vi "Compute Optimal Transition Time.vi"(8 "error in (no error)":errorcluster, 10 "optimum":T1, 11 "SV Function in":refnum<class "SV Function.lvclass">) -> (0 "error out":errorcluster, 2 "optimal transition time":dbl, 3 "SV Function out":refnum<class "SV Function.lvclass">)   [LabVIEW 2017, in "SV Function.lvclass"]
uses:
  <vilib>/addons/_NISVFA/_Generation/Signal Generation/SV Function/SV Function.lvclass
  C:/Program Files (x86)/National Instruments/LabVIEW 2017/vi.lib/addons/_NISVFA/_Generation/Signal Generation/SV Signal/SV Signal.lvclass
  <vilib>/addons/_NISVFA/_Generation/subVIs/sv_Optimum Location.ctl
  <vilib>/addons/_NISVFA/_Generation/Signal Generation/SV Signal/sv_Signal State Attribute.ctl
  <vilib>/addons/_NISVFA/_Generation/Signal Generation/SV Function/SV Function.lvclass/SV Function.ctl
  <vilib>/addons/_NISVFA/_Generation/Signal Generation/SV Signal/Read Sample Rate.vi
  <vilib>/addons/_NISVFA/_Generation/Signal Generation/SV Signal/SV Signal.lvclass
  <vilib>/addons/_NISVFA/_Generation/SoundVib_Generation.lvlib
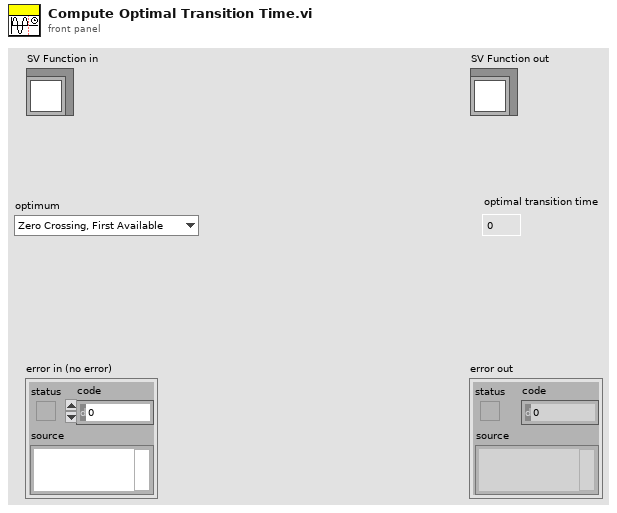
[diagram p1: front panel]
types:
  T1 = typedef "SoundVib_Generation.lvlib/sv_Optimum Location.ctl" = enum16{"Zero Crossing, First Available", "Zero Crossing, Positive Slope", "Zero Crossing, Negative Slope", "Peak or Valley", "Peak", "Valley"}
  T2 = typedef "SV Signal.lvclass/sv_Signal State Attribute.ctl" = string
  T3 = typedef "SV Signal.lvclass/sv_System Timing Model.ctl" = i64
  T4 = typedef "SV Signal.lvclass/sv_Generation State.ctl" = enum16{"Idle", "Ramp Up", "Pre-Measurement Settling", "Measurement", "Post-Measurement Settling", "Discrete Sweep Transition", "Ramp Down", "Update"}
  T5 = cluster{"system timing model":T3, "state":cluster{"RESET":bool, "generator timestamp":timestamp, "elapsed seconds":dbl, "elapsed samples":u64, "generation state":T4, "time offset at state":dbl, "samples generated at state":u64, "signal state":variant}, "duration of state":dbl, "samples remaining at state":i32}
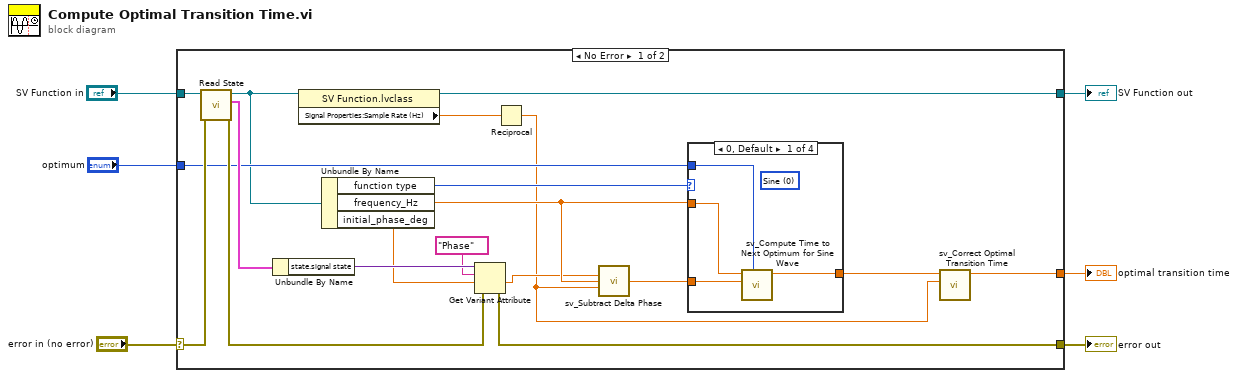
[diagram p0: block diagram]
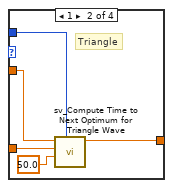
[diagram p2: hidden frame]
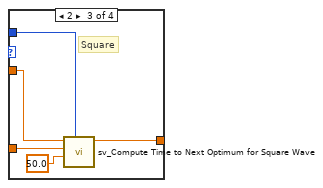
[diagram p3: hidden frame]
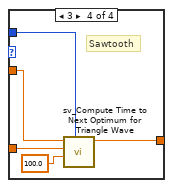
[diagram p4: hidden frame]
diagram:
  n1 = case shown="No Error" "error in (no error)" {
    selector: "error in (no error)" -> [w24 w46]
    tunnel: [w16 w46] -> w5
    tunnel: [w7 w45] -> w4
    tunnel: "SV Function in" -> [w25 w45]
    tunnel: [w13 _] -> w2
    tunnel: "optimum" -> [w20 _]
    frame No Error {
      n2 = call <vilib>:"Read State.vi"("error in (no error)"=w24, "signal configuration"=w25) -> ("error out"=w23:errorcluster, "generator state"=w22:T5, "signal configuration"=w15:refnum<class "SV Function.lvclass">)  [unwired: 7 in]
      n3 = Unbundle By Name(w22) -> ("state.signal state"=w21:variant)
      n4 = property class="SV Function.lvclass"(reference=w15) -> (reference out=w7:refnum<class "SV Function.lvclass">, "Signal Properties:Sample Rate (Hz)"=w14:dbl)  [unwired: 1 in, 1 out]
      n5 = Unbundle By Name(w15) -> ("function type"=w19:u16, "frequency_Hz"=w12:dbl, "initial_phase_deg"=w17:dbl)
      n6 = Get Variant Attribute(Variant=w21, name=T2 "Phase", default value (empty Variant)=w17, error in=w23) -> (value=w11:dbl, error out=w16:errorcluster)  [unwired: 2 out]
      n7 = Reciprocal(x=w14) -> (1/x=w8:dbl)
      n8 = call <vilib>:"sv_Subtract Delta Phase.vi"("phase in [deg]"=w11, "frequency [Hz]"=w12, "dt [s]"=w8) -> ("phase out [deg]"=w10:dbl)  [unwired: 12 in]
      n9 = case shown="0, Default" w19 {
        tunnel: w10 -> [w28 w31 w38 w43]
        tunnel: w12 -> [w29 w32 w39 w44]
        tunnel: [w26 w34 w35 w40] -> w9
        tunnel: w20 -> [w27 w33 w37 w42]
        frame 0, Default {
          (unwired) u16 0 items=["Sine", "Triangle", "Square", "Sawtooth"] ("function type")
          n10 = call <vilib>:"sv_Compute Time to Next Optimum for Sine Wave.vi"("optimum"=w27, "phase (0 °)"=w28, "frequency (997 Hz)"=w29) -> ("time to optimum [s]"=w26:dbl)  [unwired: 8 in]
        }
        frame 1 {
          # "Triangle"
          n11 = call <vilib>:"sv_Compute Time to Next Optimum for Triangle Wave.vi"("optimum"=w33, "duty cycle (50 %)"=50.0, "phase (0 °)"=w31, "frequency (997 Hz)"=w32) -> ("time to optimum [s]"=w34:dbl)  [unwired: 7 in]
        }
        frame 2 {
          # "Square"
          n12 = call <vilib>:"sv_Compute Time to Next Optimum for Square Wave.vi"("optimum"=w37, "duty cycle (50 %)"=50.0, "phase (0 °)"=w38, "frequency (997 Hz)"=w39) -> ("time to optimum [s]"=w35:dbl)  [unwired: 7 in]
        }
        frame 3 {
          # "Sawtooth"
          n13 = call <vilib>:"sv_Compute Time to Next Optimum for Triangle Wave.vi"("optimum"=w42, "duty cycle (50 %)"=100.0, "phase (0 °)"=w43, "frequency (997 Hz)"=w44) -> ("time to optimum [s]"=w40:dbl)  [unwired: 7 in]
        }
      }
      n14 = call <vilib>:"sv_Correct Optimal Transition Time.vi"("dt"=w8, "time to optimum [s]"=w9) -> ("corrected time to optimum [s]"=w13:dbl)  [unwired: 9 in]
    }
    frame Error {
    }
  }
  "error out" <- w5
  "SV Function out" <- w4
  "optimal transition time" <- w2
